vi "DrawPathToGoal.vi"(9 "Robot UTM Location":T2 {"North" format="%#_10f"; "East" format="%#_8f"}, 10 "Irons direct vector in":T1, 11 "Goal":T2 {"North" format="%#_10f"; "East" format="%#_8f"}) -> (3 "Irons direct vector out":T1)   [LabVIEW 2011]
doc: "Takes in the coordinates of the goal and the robot's current position and outputs the line between the two, including the origin, length, angle, and slope."
uses:
  2 Typedefs/UTM Location.ctl
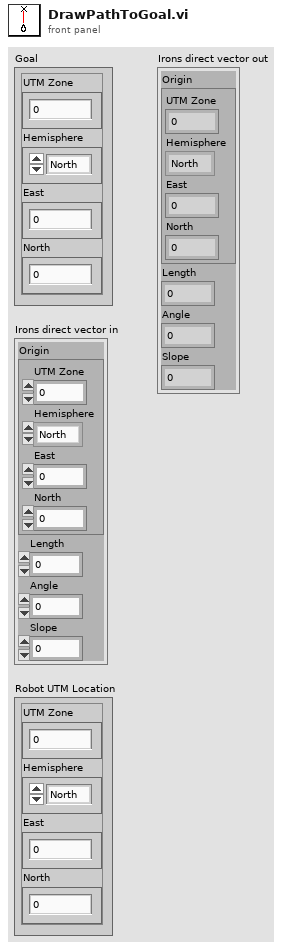
[diagram p1: front panel]
types:
  T1 = cluster{"Origin":cluster{"UTM Zone":dbl, "Hemisphere":enum16{"North", "South"}, "East":dbl, "North":dbl}, "Length":dbl, "Angle":dbl, "Slope":dbl}
  T2 = typedef "UTM Location.ctl" = cluster{"UTM Zone":dbl, "Hemisphere":enum16{"North", "South"}, "East":dbl, "North":dbl}
  T3 = typedef "heading.ctl" = dbl
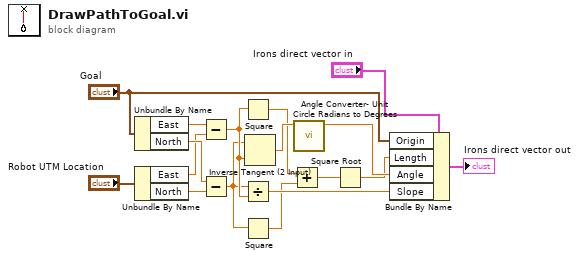
[diagram p0: block diagram]
diagram:
  n1 = Unbundle By Name("Goal") -> ("East"=w8:dbl, "North"=w10:dbl)
  n2 = Unbundle By Name("Robot UTM Location") -> ("East"=w9:dbl, "North"=w11:dbl)
  n3 = Subtract(x=w8, y=w9) -> (x-y=w17:dbl)
  n4 = Subtract(x=w10, y=w11) -> (x-y=w16:dbl)
  n5 = Square(x=w17) -> (x^2=w2:dbl)
  n6 = Divide(x=w16, y=w17) -> (x/y=w13:dbl)
  n7 = Square(x=w16) -> (x^2=w3:dbl)
  n8 = Inverse Tangent (2 Input) ("use inverse tangent\nto get heading")(1:w17, 2:w16) -> (0:w15:dbl)
  n9 = Add(x=w2, y=w3) -> (x+y=w5:dbl)
  n10 = call "Angle Converter- Unit Circle Radians to Degrees.vi"("Angle in \nUnit Circle\nRadians"=w15) -> ("Angle in \nHeading \nFormat"=w14:T3)  [unwired: 10 in]
  n11 = Square Root(x=w5) -> (sqrt(x)=w4:dbl)
  n12 = Bundle By Name(cluster="Irons direct vector in", "Origin"="Goal", "Length"=w4, "Angle"=w14, "Slope"=w13) -> (→"Irons direct vector out":T1)
